vi "Test Ordinal Dates.vi"(8 "error in":errorcluster) -> (0 "error out":errorcluster)   [LabVIEW 2013]
uses:
  <vilib>/addons/_JKI Toolkits/Caraya/classes/Test/Test.lvclass
  <vilib>/addons/_JKI Toolkits/Caraya/classes/Assert/Assert.lvclass
  <vilib>/addons/_JKI Toolkits/Caraya/classes/Assert/Assert True.vi
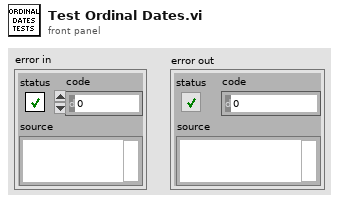
[diagram p1: front panel]
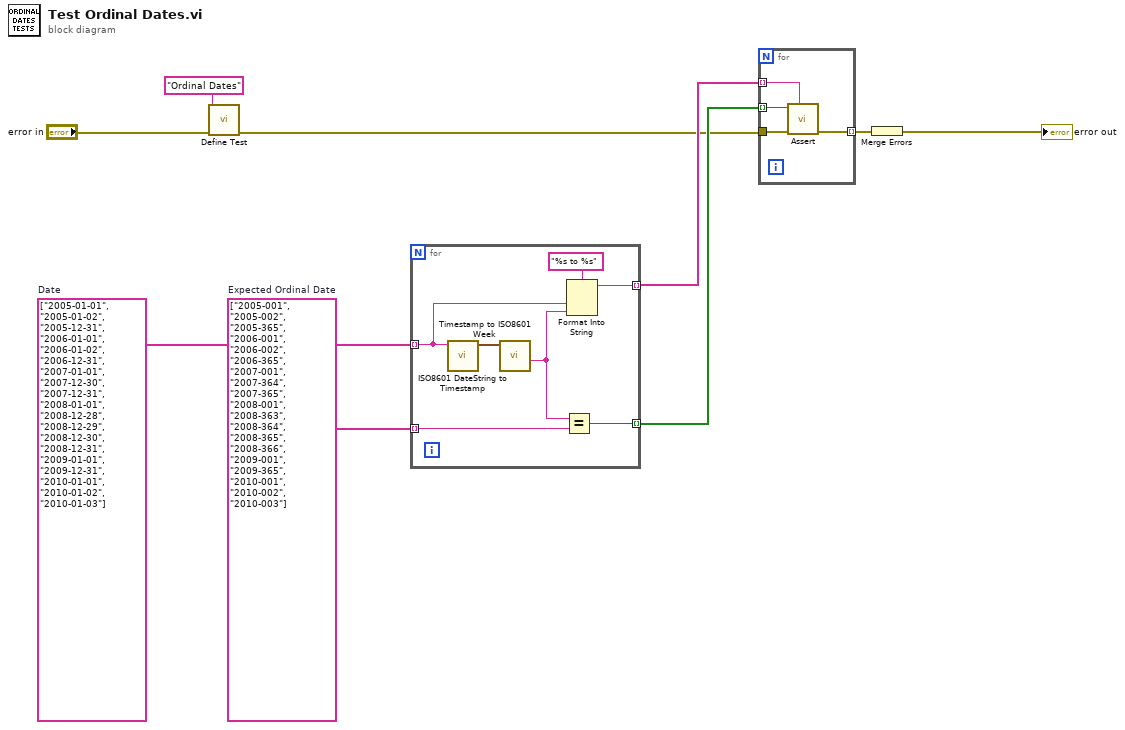
[diagram p0: block diagram]
diagram:
  w8 = string[] ["2005-01-01", "2005-01-02", "2005-12-31", "2006-01-01", "2006-01-02", "2006-12-31", "2007-01-01", "2007-12-30", "2007-12-31", "2008-01-01", "2008-12-28", "2008-12-29", "2008-12-30", "2008-12-31", "2009-01-01", "2009-12-31", "2010-01-01", "2010-01-02", "2010-01-03"]  # Date
  w9 = string[] ["2005-001", "2005-002", "2005-365", "2006-001", "2006-002", "2006-365", "2007-001", "2007-364", "2007-365", "2008-001", "2008-363", "2008-364", "2008-365", "2008-366", "2009-001", "2009-365", "2010-001", "2010-002", "2010-003"]  # Expected Ordinal Date
  n1 = call <vilib>:"Define Test.vi"("error in (no error)"="error in", "Label (VI Title)"="Ordinal Dates") -> ("error out"=w2:errorcluster)  [unwired: 8 in, 1 out]
  n2 = for {
    tunnel: w9 -> [w16] mode=indexing
    tunnel: w8 -> [w11] mode=indexing
    tunnel: [w13] -> w4 mode=indexing
    tunnel: [w12] -> w5 mode=indexing
    n3 = call "ISO8601 DateString to Timestamp.vi"("ISO8601 String"=w11) -> ("Timestamp"=w15:timestamp)  [unwired: 8 in, 2 out]
    n4 = call "Timestamp to ISO8601 Week.vi"("Timestamp (now)"=w15) -> ("ISO8601 Ordinal Date"=w10:string)  [unwired: 8 in, 2 out]
    n5 = Equal?(x=w10, y=w16) -> (x = y?=w12:bool)
    n6 = Format Into String(format string="%s to %s" ("Label (VI Title)"), w11, w10) -> (resulting string=w13:string)  [unwired: 2 in, 1 out]
  }
  n7 = for {
    tunnel: w2 -> [w20]
    tunnel: [w19] -> w7 mode=indexing
    tunnel: w4 -> [w18] mode=indexing
    tunnel: w5 -> [w17] mode=indexing
    n8 = call-poly <vilib>:"Assert.vi"("Label"=w18, "error in (no error)"=w20, "True?"=w17) -> ("error out"=w19:errorcluster)  [unwired: 7 in, 1 out]
  }
  n9 = Merge Errors(w7) -> (→"error out":errorcluster)
